vi "Actor Core.vi"(8 "error in":cluster{"状态":bool, "代码":i32, "源":string} caption="错误输入", 11 "Alpha":refnum<class "Alpha.lvclass"> caption="DNL_Alpha") -> (0 "error out":cluster{"状态":bool, "代码":i32, "源":string} caption="错误输出", 3 "操作者输出":refnum<class "Actor.lvclass">)   [LabVIEW 2013, in "Alpha操作者.lvlib" / "Alpha.lvclass"]
doc: "Actor Core.vi包含操作者的主要消息处理循环。操作者通常位于该循环中，在各种消息到达时对消息进行处理。如Do.vi消息返回任何错误，该循环将停止运行，错误代码43将被作为“无错误停止”的标准信号发送给调用方。如需更改上述行为，可在子孙类的Handle Error.vi中对该部分逻辑进行重写。"
uses:
  Alpha.lvclass
  <vilib>/ActorFramework/Actor/Actor.lvclass
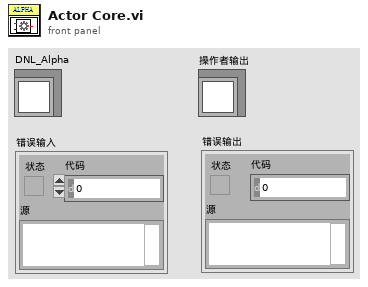
[diagram p1: front panel]
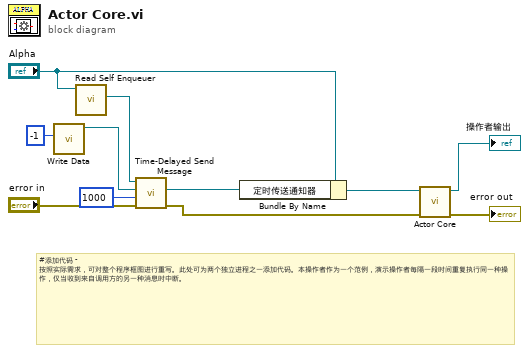
[diagram p0: block diagram]
diagram:
  # "#添加代码 - 按照实际需求，可对整个程序框图进行重写。此处可为两个独立进程之一添加代码。本操作者作为一个范例，演示操作者每隔一段时间重复执行同一种操作，仅当收到来自调用方的另一种消息时中断。"
  n1 = call "Write Data.vi"("数据"=-1 ("Data")) -> ("Alpha任务消息输出"=w2:refnum<class "Alpha任务消息.lvclass">)  [unwired: 10 in]
  n2 = call <vilib>:"Read Self Enqueuer.vi"("Actor"="Alpha") -> ("Self Enqueuer"=w9:refnum<class "Message Enqueuer.lvclass">)  [unwired: 10 in]
  n3 = call <vilib>:"Time-Delayed Send Message.vi"("error in (no error)"="error in", "Milliseconds To Wait"=1000, "Message"=w2, "Message Enqueuer"=w9) -> ("error out"=w3:errorcluster, "Delivery Notifier"=w5:refnum<notifier>)  [unwired: 6 in]
  n4 = Bundle By Name(cluster="Alpha", "定时传送通知器"=w5) -> (w6:refnum<class "Alpha.lvclass">)
  n5 = call-parent "Actor Core.vi"("error in"=w3, "Actor in"=w6) -> ("error out"=→"error out":errorcluster, "Actor out"=→"操作者输出":refnum<class "Actor.lvclass">)  [unwired: 8 in]
